vi "ScalingLockLogic.vi"   [LabVIEW 2016]
uses:
  <vilib>/Rock Robotics/WPI/Solenoid/WPI_SolenoidValue.ctl
  <vilib>/Rock Robotics/WPI/Solenoid/WPI_SolenoidSetEnum.vi
  Robot Global Data.vi
  <vilib>/Rock Robotics/WPI/Solenoid/Deprecated/WPI_SolenoidGetBool.vi
  <vilib>/Rock Robotics/WPI/Solenoid/Deprecated/WPI_SolenoidSetBool.vi
  <vilib>/Rock Robotics/Network Tables/NT Write Boolean.vi
types:
  T1 = typedef "WPI_SolenoidValue.ctl" = enum16{"Off", "On", "Forward", "Reverse"}
  T2 = typedef "WPI_SolenoidDevRef.ctl" = cluster{"DevStatus":errorcluster, "Pneumatics Control Module":u8, "Forward Solenoid Channel":T3, "Reverse Solenoid Channel":T3}
  T3 = typedef "WPI_SolenoidChannel.ctl" = enum8{"Solenoid 0", "Solenoid 1", "Solenoid 2", "Solenoid 3", "Solenoid 4", "Solenoid 5", "Solenoid 6", "Solenoid 7", "Invalid"}
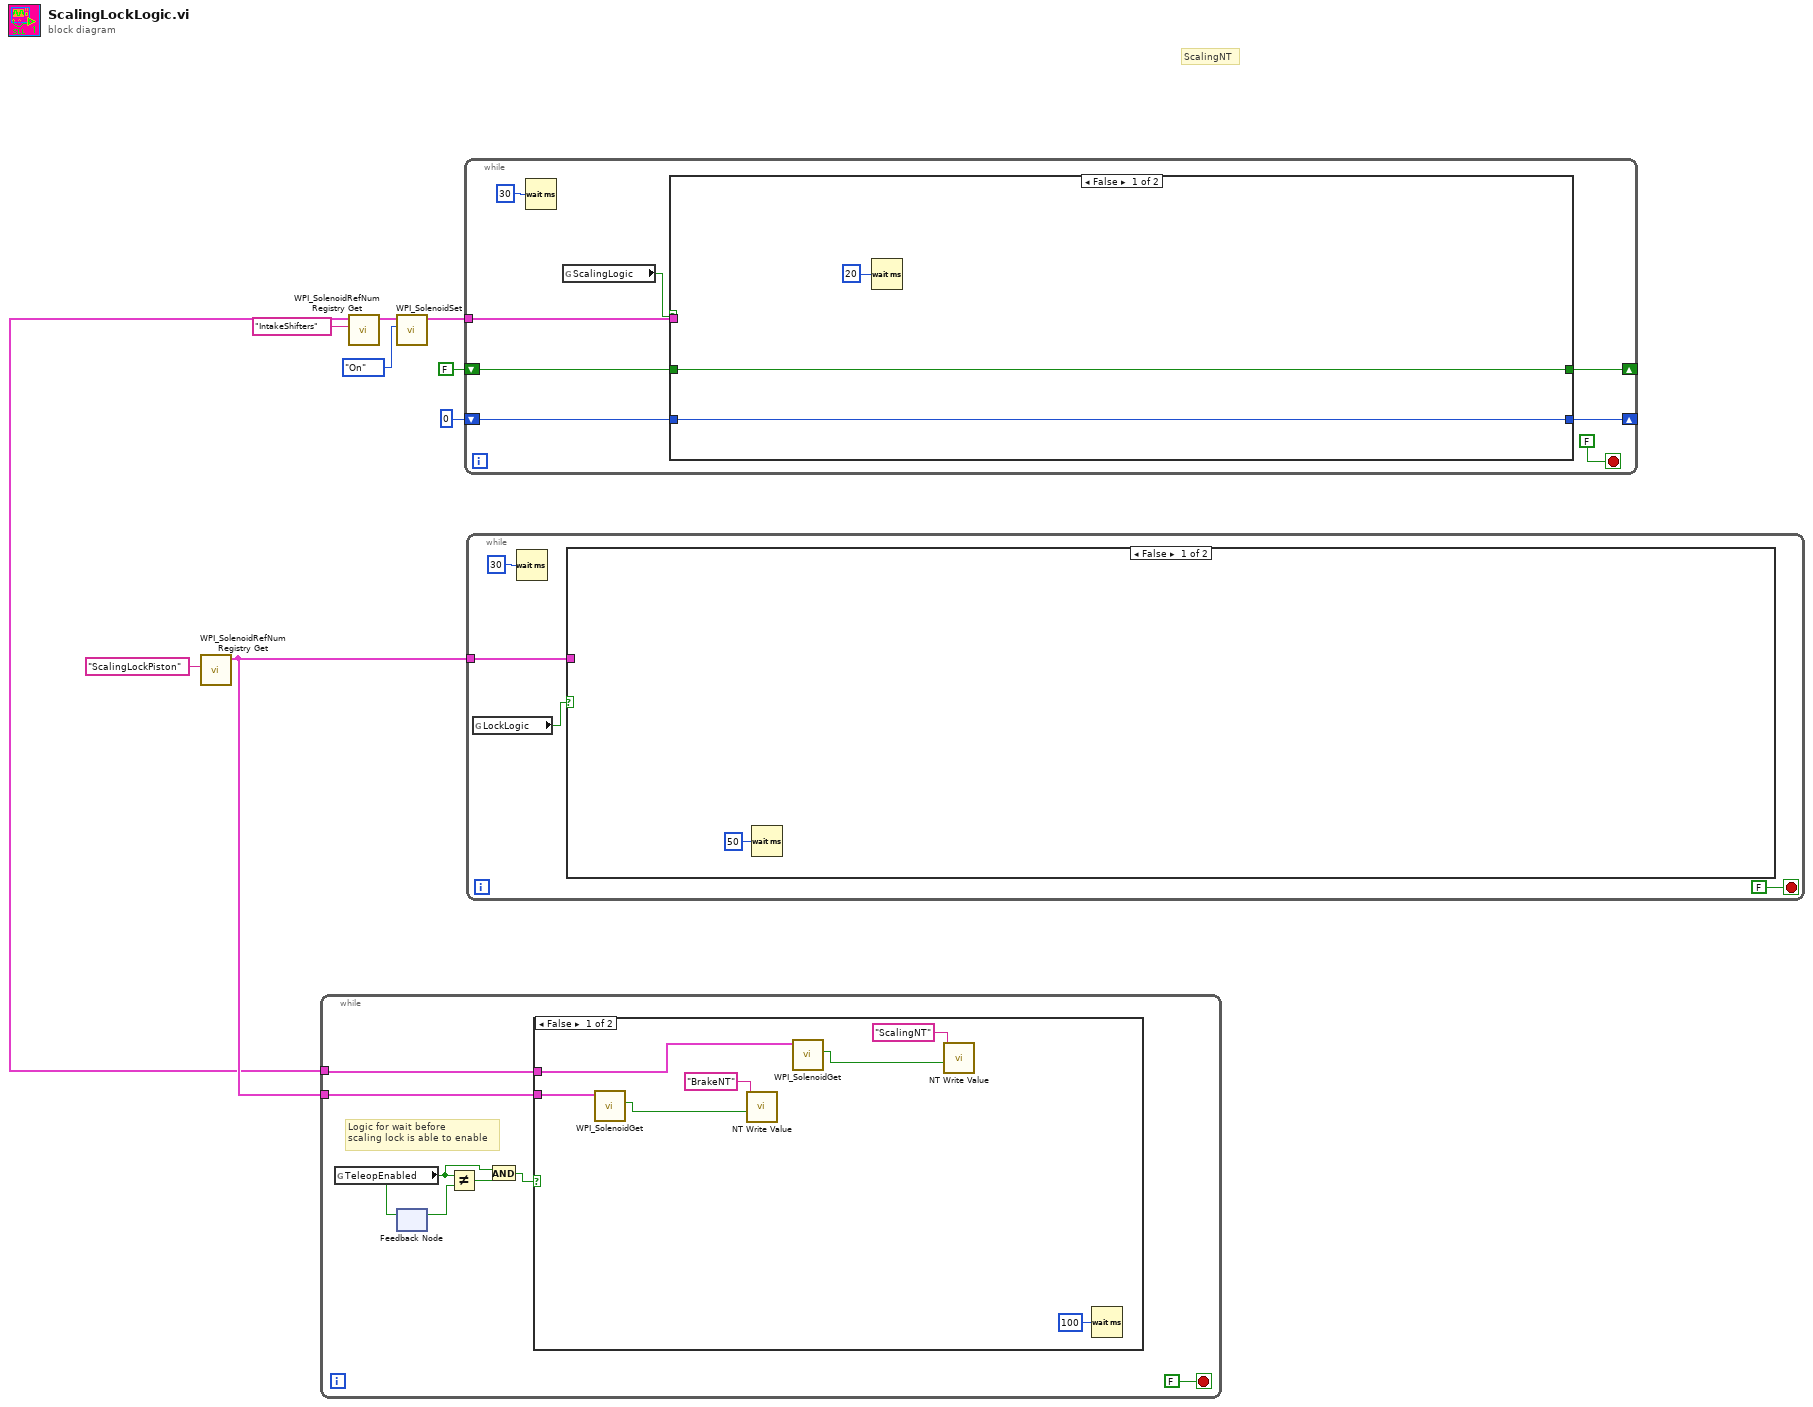
[diagram p0: block diagram]
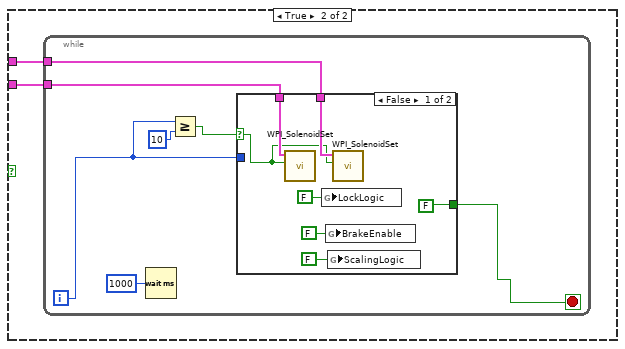
[diagram p2: hidden frame]
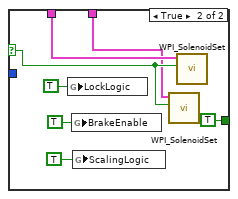
[diagram p3: hidden frame]
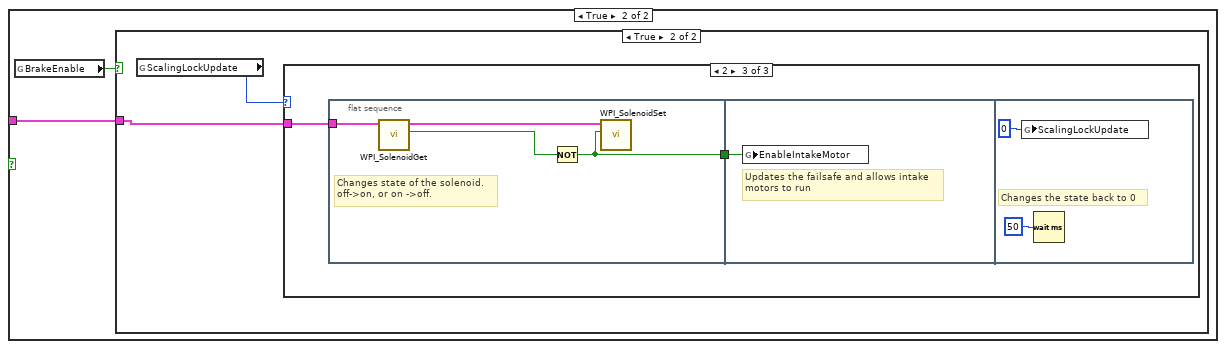
[diagram p4: hidden frame]
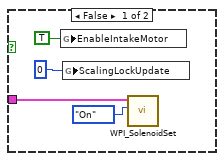
[diagram p5: hidden frame]
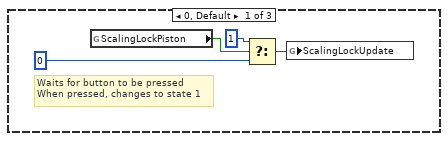
[diagram p6: hidden frame]
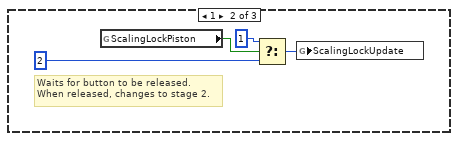
[diagram p7: hidden frame]
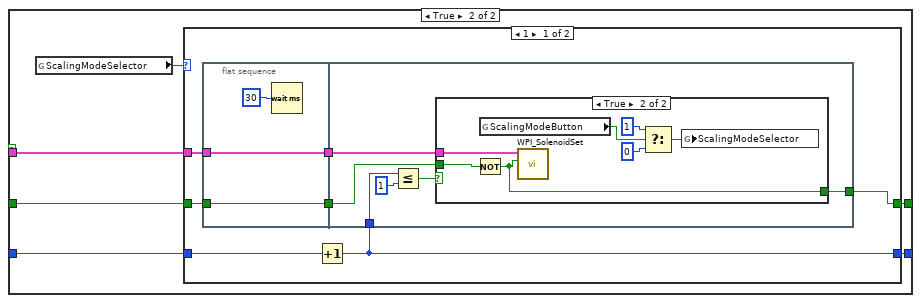
[diagram p8: hidden frame]
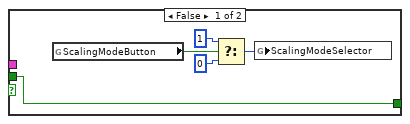
[diagram p9: hidden frame]
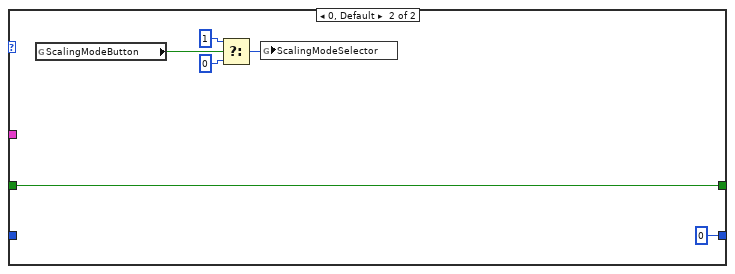
[diagram p10: hidden frame]
diagram:
  # "ScalingNT"
  n1 = call <vilib>:"WPI_SolenoidRefNum Registry Get.vi"("refnum name"="ScalingLockPiston") -> ("SolenoidDevRef"=w3:T2)  [unwired: 9 in, 1 out]
  n2 = call <vilib>:"WPI_SolenoidRefNum Registry Get.vi"("refnum name"="IntakeShifters") -> ("SolenoidDevRef"=w5:T2)  [unwired: 9 in, 1 out]
  n3 = call-poly <vilib>:"WPI_SolenoidSet.vi"("Value"=WPI_SolenoidValue."On", "SolenoidDevRef"=w5) -> ("SolenoidDevRef"=w1:T2)  [unwired: 8 in, 1 out]
  n4 = while {
    tunnel: w3 -> [w15]
    tunnel: w1 -> [w9]
    stop <- FALSE stop-if-true
    # "Logic for wait before \nscaling lock is able to enable"
    n5 = global read "Robot Global Data.vi" "TeleopEnabled"() -> (w11:bool)
    n6 = feedback-in #1(w11) -> ()
    n7 = feedback #1() -> (w13:bool)  [unwired: 1 in]
    n8 = Not Equal?(x=w11, y=w13) -> (x != y?=w12:bool)
    n9 = And(x=w11, y=w12) -> (x .and. y?=w10:bool)
    n10 = case shown="False" w10 {
      tunnel: w15 -> [w16 w24]
      tunnel: w9 -> [w18 w23]
      frame False {
        n11 = call-poly <vilib>:"WPI_SolenoidGet.vi"("SolenoidDevRef"=w16) -> ("Value"=w17:bool)  [unwired: 8 in, 2 out]
        n12 = call-poly <vilib>:"NT Write Value.vi"("Boolean"=w17, "Name"="BrakeNT") -> ()  [unwired: 9 in, 1 out]
        n13 = call-poly <vilib>:"WPI_SolenoidGet.vi"("SolenoidDevRef"=w18) -> ("Value"=w19:bool)  [unwired: 8 in, 2 out]
        n14 = call-poly <vilib>:"NT Write Value.vi"("Boolean"=w19, "Name"="ScalingNT") -> ()  [unwired: 9 in, 1 out]
        n15 = Wait (ms)(milliseconds to wait=u32 100) -> ()  [unwired: 1 out]
      }
      frame True {
        n16 = while {
          tunnel: w24 -> [w27]
          tunnel: w23 -> [w25]
          i -> [w29]
          stop <- w26 stop-if-true
          n17 = Wait (ms)(milliseconds to wait=u32 1000) -> ()  [unwired: 1 out]
          n18 = Greater Or Equal?(x=w29, y=10) -> (x >= y?=w30:bool)
          n19 = case shown="False" w30 {
            selector: w30 -> [w32 w40]
            tunnel: w29 -> [_ _]
            tunnel: w27 -> [w35 w44]
            tunnel: [FALSE TRUE] -> w26
            tunnel: w25 -> [w33 w39]
            frame False {
              n20 = call-poly <vilib>:"WPI_SolenoidSet.vi"("Value"=w32, "SolenoidDevRef"=w35) -> ()  [unwired: 8 in, 2 out]
              n21 = global write "Robot Global Data.vi" "LockLogic"(FALSE ("LockLogic")) -> ()
              n22 = global write "Robot Global Data.vi" "BrakeEnable"(FALSE ("BrakeEnable")) -> ()
              n23 = global write "Robot Global Data.vi" "ScalingLogic"(FALSE ("BrakeEnable")) -> ()
              n24 = call-poly <vilib>:"WPI_SolenoidSet.vi"("Value"=w32, "SolenoidDevRef"=w33) -> ()  [unwired: 8 in, 2 out]
            }
            frame True {
              n25 = global write "Robot Global Data.vi" "LockLogic"(TRUE ("LockLogic")) -> ()
              n26 = global write "Robot Global Data.vi" "BrakeEnable"(TRUE ("BrakeEnable")) -> ()
              n27 = global write "Robot Global Data.vi" "ScalingLogic"(TRUE ("BrakeEnable")) -> ()
              n28 = call-poly <vilib>:"WPI_SolenoidSet.vi"("Value"=w40, "SolenoidDevRef"=w39) -> ()  [unwired: 8 in, 2 out]
              n29 = call-poly <vilib>:"WPI_SolenoidSet.vi"("Value"=w40, "SolenoidDevRef"=w44) -> ()  [unwired: 8 in, 2 out]
            }
          }
        }
      }
    }
  }
  n30 = while {
    shift-right: [w52] -> _
    shift-left: FALSE -> [w50]
    tunnel: w1 -> [w49]
    shift-right: [w48] -> _
    shift-left: 0 -> [w47]
    stop <- FALSE stop-if-true
    n31 = Wait (ms)(milliseconds to wait=u32 30) -> ()  [unwired: 1 out]
    n32 = global read "Robot Global Data.vi" "ScalingLogic"() -> (w46:bool)
    n33 = case shown="False" w46 {
      tunnel: [w56 w61] -> w52
      tunnel: w50 -> [w56 w60]
      tunnel: w49 -> [_ w59]
      tunnel: [w55 w58] -> w48
      tunnel: w47 -> [w55 w57]
      frame False {
        n34 = Wait (ms)(milliseconds to wait=u32 20) -> ()  [unwired: 1 out]
      }
      frame True {
        n35 = global read "Robot Global Data.vi" "ScalingModeSelector"() -> (w62:i32)
        n36 = case shown="1" w62 {
          tunnel: [w63 w92] -> w61
          tunnel: w60 -> [w68 w92]
          tunnel: w59 -> [w67 _]
          tunnel: [w65 0] -> w58
          tunnel: w57 -> [w66 _]
          frame 1 {
            n37 = flat-sequence {
              tunnel: [w71] -> w69
              tunnel: w68 -> [w71]
              tunnel: w67 -> [w70]
              tunnel: [w70] -> w64
              tunnel: w69 -> [w74]
              tunnel: w65 -> [w76]
              tunnel: w64 -> [w75]
              tunnel: [w73] -> w63
              frame #0 {
                n38 = Wait (ms)(milliseconds to wait=u32 30) -> ()  [unwired: 1 out]
              }
              frame #1 {
                n39 = Less Or Equal?(x=w76, y=1) -> (x <= y?=w78:bool)
                n40 = case shown="True" w78 {
                  tunnel: w74 -> [w79 w90]
                  tunnel: w75 -> [_ w85]
                  tunnel: [w79 w84] -> w73
                  frame False {
                    n41 = global read "Robot Global Data.vi" "ScalingModeButton"() -> (w80:bool)
                    n42 = Select(t=1, s=w80, f=0) -> (s? t:f=w82:i32)
                    n43 = global write "Robot Global Data.vi" "ScalingModeSelector"(w82) -> ()
                  }
                  frame True {
                    n44 = Not(x=w90) -> (.not. x?=w84:bool)
                    n45 = global read "Robot Global Data.vi" "ScalingModeButton"() -> (w89:bool)
                    n46 = call-poly <vilib>:"WPI_SolenoidSet.vi"("Value"=w84, "SolenoidDevRef"=w85) -> ()  [unwired: 8 in, 2 out]
                    n47 = Select(t=1, s=w89, f=0) -> (s? t:f=w87:i32)
                    n48 = global write "Robot Global Data.vi" "ScalingModeSelector"(w87) -> ()
                  }
                }
              }
            }
            n49 = Increment(x=w66) -> (x+1=w65:i32)
          }
          frame 0, Default {
            n50 = global read "Robot Global Data.vi" "ScalingModeButton"() -> (w96:bool)
            n51 = Select(t=1, s=w96, f=0) -> (s? t:f=w94:i32)
            n52 = global write "Robot Global Data.vi" "ScalingModeSelector"(w94) -> ()
          }
        }
      }
    }
  }
  n53 = while {
    tunnel: w3 -> [w99]
    stop <- FALSE stop-if-true
    n54 = global read "Robot Global Data.vi" "LockLogic"() -> (w97:bool)
    n55 = Wait (ms)(milliseconds to wait=u32 30) -> ()  [unwired: 1 out]
    n56 = case shown="False" w97 {
      tunnel: w99 -> [_ w102]
      frame False {
        n57 = Wait (ms)(milliseconds to wait=u32 50) -> ()  [unwired: 1 out]
      }
      frame True {
        n58 = global read "Robot Global Data.vi" "BrakeEnable"() -> (w103:bool)
        n59 = case shown="True" w103 {
          tunnel: w102 -> [w104 w108]
          frame False {
            n60 = global write "Robot Global Data.vi" "EnableIntakeMotor"(TRUE ("EnableIntakeMotor")) -> ()
            n61 = global write "Robot Global Data.vi" "ScalingLockUpdate"(0) -> ()
            n62 = call-poly <vilib>:"WPI_SolenoidSet.vi"("Value"=WPI_SolenoidValue."On", "SolenoidDevRef"=w104) -> ()  [unwired: 8 in, 2 out]
          }
          frame True {
            n63 = global read "Robot Global Data.vi" "ScalingLockUpdate"() -> (w109:i32)
            n64 = case shown="2" w109 {
              tunnel: w108 -> [_ _ w118]
              frame 0, Default {
                # "Waits for button to be pressed\nWhen pressed, changes to state 1"
                n65 = global read "Robot Global Data.vi" "ScalingLockPiston"() -> (w113:bool)
                n66 = Select(t=1, s=w113, f=0) -> (s? t:f=w110:i32)
                n67 = global write "Robot Global Data.vi" "ScalingLockUpdate"(w110) -> ()
              }
              frame 1 {
                # "Waits for button to be released.\nWhen released, changes to stage 2."
                n68 = global read "Robot Global Data.vi" "ScalingLockPiston"() -> (w117:bool)
                n69 = Select(t=1, s=w117, f=2) -> (s? t:f=w114:i32)
                n70 = global write "Robot Global Data.vi" "ScalingLockUpdate"(w114) -> ()
              }
              frame 2 {
                n71 = flat-sequence {
                  tunnel: [w120] -> w119
                  tunnel: w118 -> [w122]
                  tunnel: w119 -> [w124]
                  frame #0 {
                    # "Changes state of the solenoid.\noff->on, or on ->off."
                    n72 = call-poly <vilib>:"WPI_SolenoidGet.vi"("SolenoidDevRef"=w122) -> ("Value"=w121:bool, "SolenoidDevRef"=w123:T2)  [unwired: 8 in, 1 out]
                    n73 = Not(x=w121) -> (.not. x?=w120:bool)
                    n74 = call-poly <vilib>:"WPI_SolenoidSet.vi"("Value"=w120, "SolenoidDevRef"=w123) -> ()  [unwired: 8 in, 2 out]
                  }
                  frame #1 {
                    # "Updates the failsafe and allows intake\nmotors to run"
                    n75 = global write "Robot Global Data.vi" "EnableIntakeMotor"(w124) -> ()
                  }
                  frame #2 {
                    # "Changes the state back to 0"
                    n76 = global write "Robot Global Data.vi" "ScalingLockUpdate"(0) -> ()
                    n77 = Wait (ms)(milliseconds to wait=u32 50) -> ()  [unwired: 1 out]
                  }
                }
              }
            }
          }
        }
      }
    }
  }
